vi "SMC_SendCommand.vi"(8 "error in (no error)":errorcluster, 11 "Command":string) -> (0 "error out":errorcluster, 3 "Answer":string)   [LabVIEW 2015]
uses:
  SMC_SubVIs.llb/SMC_ManagerMode.ctl
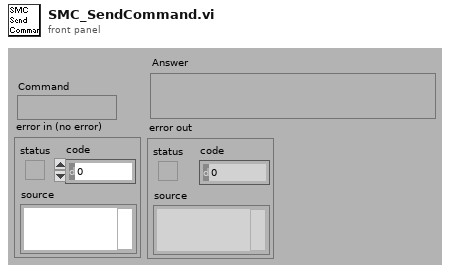
[diagram p1: front panel]
types:
  T1 = typedef "SMC_ManagerMode.ctl" = enum16{"Init", "Get", "SetPosition", "SetStatus", "SetMoving", "SetControllerNr"}
  T2 = typedef "SMC Paras.ctl" = cluster{"VENUS Language":T3, "Number of Axis":u8, "Controller Nr":u8, "Simulation":bool}
  T3 = typedef "VENUSNr.ctl" = enum16{"VENUS 2", "VENUS 1"}
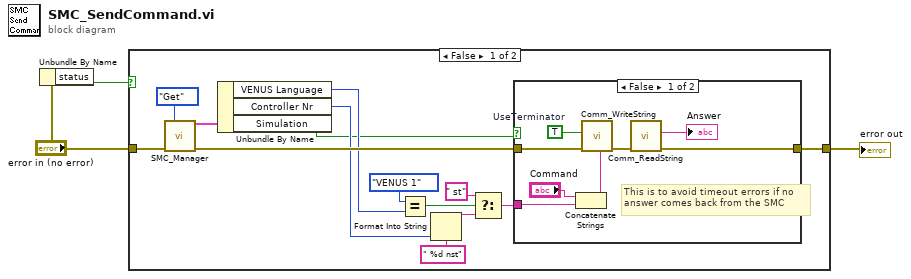
[diagram p0: block diagram]
diagram:
  n1 = Unbundle By Name("error in (no error)") -> ("status"=w2:bool)
  n2 = case shown="False" w2 {
    tunnel: "error in (no error)" -> [w14 w27]
    tunnel: [w16 w27] -> w1
    frame False {
      n3 = call "SMC_Manager.vi"("Mode"=SMC_ManagerMode."Get", "error in (no error)"=w14) -> ("SMC Parameter Out"=w6:T2, "error out"=w15:errorcluster)  [unwired: 9 in, 3 out]
      n4 = Unbundle By Name(w6) -> ("VENUS Language"=w7:T3, "Controller Nr"=w5:u8, "Simulation"=w4:bool)
      n5 = Equal?(x=enum16{"VENUS 2", "VENUS 1"}."VENUS 1" ("y"), y=w7) -> (x = y?=w11:bool)
      n6 = Format Into String(format string=" %d nst" ("Format String"), w5) -> (resulting string=w8:string)  [unwired: 2 in, 1 out]
      n7 = Select(t=" st", s=w11, f=w8) -> (s? t:f=w13:string)
      n8 = case shown="False" w4 {
        tunnel: [w23 w26] -> w16
        tunnel: w15 -> [w22 w26]
        tunnel: w13 -> [w19 _]
        frame False {
          w18 = TRUE  # UseTerminator
          # "This is to avoid timeout errors if no \nanswer comes back from the SMC"
          n9 = Concatenate Strings("Command", w19) -> (w21:string)
          n10 = call "Comm_WriteString.vi"("string to write"=w21, "error in (no error)"=w22, "UseTerminator"=w18) -> ("error out"=w24:errorcluster)  [unwired: 8 in]
          n11 = call "Comm_ReadString.vi"("error in (no error)"=w24) -> ("error out"=w23:errorcluster, "Answer"=→"Answer":string)  [unwired: 9 in]
        }
        frame True {
        }
      }
    }
    frame True {
      # "Error, do nothing"
    }
  }
  "error out" <- w1
